vi "Initialize and Calibrate.vi"() -> (0 "Calibrated":bool, 3 "IO Cluster":T1={"Error"={"status"=FALSE, "code"=0, "source"=""}, "Encoder Calibration Values"=[22, 216], "Update Calibration"=FALSE, "JPEG Resolutions"=3, "Raw Resolutions"=1, "Image Mode"=enum."RAW Gray Scale", "FPGA Ref"=refnum} {"JPEG Resolutions" items=["160x128"=3, "320x240"=5, "640x480"=7]; "Raw Resolutions" items=["80x60"=1, "160x120"=3, "128x128"=9, "128x96"=11]})   [LabVIEW 2018]
uses:
  QNET MS IO Cluster.ctl
  <vilib>/Platform/TimedLoop/XDataNode/timing_clust.ctl
  <vilib>/Platform/TimedLoop/XDataNode/nitl_modes.ctl
  <vilib>/Platform/TimedLoop/XDataNode/wakeup.ctl
  <extravilib>/ChannelInstances/Tag-c(a[.](dbl),a[.](c(c(sgl,sgl),sgl,sgl,sgl,a[.](c(sgl,sgl)))))/Read With Abort.vi
  <extravilib>/ChannelInstances/Tag-bool/Write With Abort.vi
  <extravilib>/ChannelInstances/Tag-bool/Read With Abort.vi
  <extravilib>/ChannelInstances/Tag-c(a[.](dbl),a[.](c(c(sgl,sgl),sgl,sgl,sgl,a[.](c(sgl,sgl)))))/Write With Abort.vi
  <extravilib>/ChannelInstances/Tag-c(a[.](dbl),a[.](c(c(sgl,sgl),sgl,sgl,sgl,a[.](c(sgl,sgl)))))/Instantiate.vi
  <extravilib>/ChannelInstances/Tag-bool/Instantiate.vi
  <extravilib>/ChannelInstances/Tag-bool/EndpointRead.vi
  <extravilib>/ChannelInstances/Tag-c(a[.](dbl),a[.](c(c(sgl,sgl),sgl,sgl,sgl,a[.](c(sgl,sgl)))))/Endpoint.vi
  <extravilib>/ChannelInstances/Tag-c(a[.](dbl),a[.](c(c(sgl,sgl),sgl,sgl,sgl,a[.](c(sgl,sgl)))))/EndpointRead.vi
  <extravilib>/ChannelInstances/Tag-bool/Endpoint.vi
  <vilib>/Platform/TimedLoop/XDataNode/XDataNode.xnode
  <extravilib>/ChannelInstances/Tag-bool.lvlib
  <vilib>/Platform/TimedLoop/XDataNode/XDNodeRunTimeDep.lvlib
  <extravilib>/ChannelInstances/Tag-c(a[.](dbl),a[.](c(c(sgl,sgl),sgl,sgl,sgl,a[.](c(sgl,sgl))))).lvlib
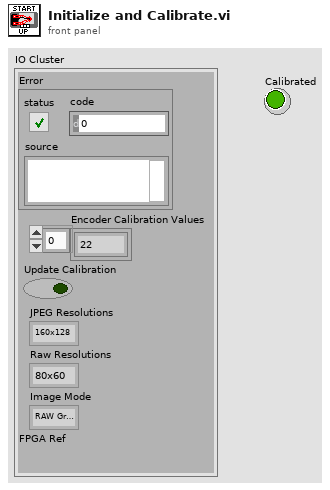
[diagram p1: front panel]
types:
  T1 = typedef "QNET MS IO Cluster.ctl" = cluster{"Error":errorcluster, "Encoder Calibration Values":i32[], "Update Calibration":bool, "JPEG Resolutions":u16, "Raw Resolutions":u16, "Image Mode":enum16{"RAW RGB", "RAW Gray Scale", "JPEG"}, "FPGA Ref":refnum<k20>}
  T2 = typedef "IMAQ Image.ctl" = refnum<image>
  T3 = typedef "XDNodeRunTimeDep.lvlib/timing_clust.ctl" = cluster{"Expected End [f-1]":u64, "Actual End [f-1]":u64, "Finished Late? [f-1]":bool, "Expected End [i-1]":u64, "Actual End [i-1]":u64, "Finished Late? [i-1]":bool, "Expected Start [i]":u64, "Actual Start [i]":u64, "Expected Start [f]":u64, "Actual Start [f]":u64, "Source Name":string, "Structure Name":string, "Period":i64, "Deadline":i64, "Offset":i64, "Start":i64, "Priority":i32, "Timeout":i32, "Mode":T4, "Wakeup Reason":T5, "Error":errorcluster, "Source Type":string, "Secondary Source Type":string, "Global End Time":u64, "Global Start Time":u64, "Frame Duration":u64, "Iteration Duration":u64, "Assigned CPU":i32, "I/O Scan Engine Mode":u32}
  T4 = typedef "XDNodeRunTimeDep.lvlib/nitl_modes.ctl" = enum32{"No Change", "Process missed periods, maintain original phase", "Discard missed periods, maintain original phase", "Process missed periods, ignore original phase", "Discard missed periods, ignore original phase"}
  T5 = typedef "XDNodeRunTimeDep.lvlib/wakeup.ctl" = enum32{"Normal", "Aborted", "Asynchronous wakeup", "Timing source error", "Timed loop error", "Timeout"}
  T6 = cluster{"Joint Coordinates (rad)":dbl[], "Matches (pixel)":cluster{"Position":cluster{"x":sgl, "y":sgl}, "Angle":sgl, "Scale":sgl, "Score":sgl, "Bounding Box":cluster{"x":sgl, "y":sgl}[]}[]}
  T7 = typedef "Tag-c(a[.](dbl),a[.](c(c(sgl,sgl),sgl,sgl,sgl,a[.](c(sgl,sgl))))).lvlib/))Channel.ctl" = refnum<queue>
  T8 = typedef "Tag-bool.lvlib/))Channel.ctl" = refnum<queue>
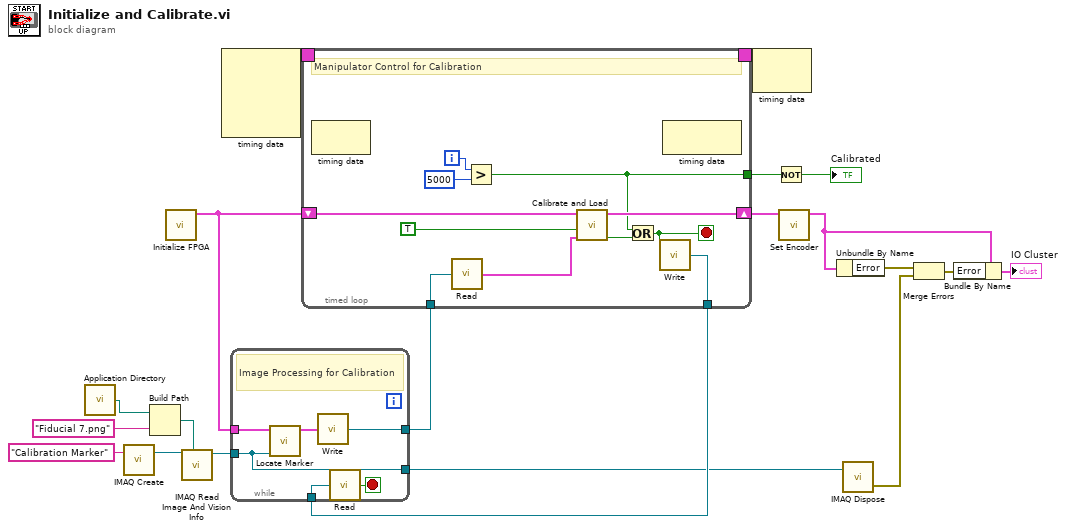
[diagram p0: block diagram]
diagram:
  n1 = call <vilib>:"Application Directory.vi"() -> ("Application Directory"=w11:path)
  n2 = call "IMAQ Create"("Image Name"="Calibration Marker") -> ("New Image"=w9:T2)  [unwired: 4 in, 1 out]
  n3 = Build Path(base path=w11, name or relative path="Fiducial 7.png") -> (appended path=w8:path)
  n4 = call "Initialize FPGA.vi"() -> ("IO Cluster Out"=w18:T1)  [unwired: 3 in]
  n5 = call "IMAQ Read Image And Vision Info"("File Path"=w8, "Image"=w9) -> ("Image Out"=w7:T2)  [unwired: 7 in, 2 out]
  n6 = node-c288() -> (w20:T3)  [unwired: 4 in]
  n7 = while {
    tunnel: w18 -> [w23]
    tunnel: w17 -> [w26]
    tunnel: w7 -> [w24]
    tunnel: [w24] -> w6
    tunnel: [w21] -> w2
    stop <- w25 stop-if-true
    # "Image Processing for Calibration"
    n8 = call "Locate Marker.vi"("Marker Image"=w24, "IO Cluster In"=w23) -> ("Marker Calibration Cluster"=w22:T6)  [unwired: 8 in, 1 out]
    n9 = call <extravilib>:"Write.vi"("element"=w22) -> ("channel"=w21:T7)  [unwired: 1 out]
    n10 = call <extravilib>:"Read.vi"("channel"=w26) -> ("element"=w25:bool)  [unwired: 1 in, 1 out]
  }
  n11 = timed-loop {
    shift-right: [w36] -> w1
    shift-left: w18 -> [w33]
    timing: w20 -> [_]
    timing-out: [_] -> w19
    tunnel: [w37] -> w17
    tunnel: [w30] -> w4
    tunnel: w2 -> [w28]
    i -> [w32]
    stop <- w35 stop-if-true
    # "Manipulator Control for Calibration"
    n12 = node-c288() -> ()  [unwired: 1 in, 1 out]
    n13 = call <extravilib>:"Read.vi"("channel"=w28) -> ("element"=w27:T6)  [unwired: 1 in, 1 out]
    n14 = Greater?(x=w32, y=5000) -> (0:w30:bool)
    n15 = call "Calibrate and Load.vi"("Calibration Cluster"=w27, "Always Calibrate"=TRUE, "IO Cluster In"=w33) -> ("Exit Loop"=w34:bool, "IO Cluster Out"=w36:T1)  [unwired: 6 in, 1 out]
    n16 = Or(x=w30, y=w34) -> (x .or. y?=w35:bool)
    n17 = call <extravilib>:"Write.vi"("element"=w35) -> ("channel"=w37:T8)  [unwired: 1 out]
    n18 = node-c288() -> ()  [unwired: 1 in, 1 out]
  }
  n19 = node-c288(w19) -> ()  [unwired: 1 out]
  n20 = Not(x=w4) -> (.not. x?=→"Calibrated":bool)
  n21 = call "Set Encoder.vi"("IO Cluster In"=w1) -> ("IO Cluster Out"=w14:T1)  [unwired: 10 in]
  n22 = Unbundle By Name(w14) -> ("Error"=w15:errorcluster)
  n23 = call "IMAQ Dispose"("Image"=w6) -> ("error out"=w5:errorcluster)  [unwired: 5 in]
  n24 = Merge Errors(w15, w5) -> (w16:errorcluster)
  n25 = Bundle By Name(cluster=w14, "Error"=w16) -> (→"IO Cluster":T1)
